vi "default zero array.vi"(7 "Array":dbl[](array[numeric]), 9 "frekans size":dbl, 10 "size":dbl, 11 "control hz array":dbl[][](array[numeric])) -> (3 "output array":dbl[][](array[numeric]))   [LabVIEW 2014]
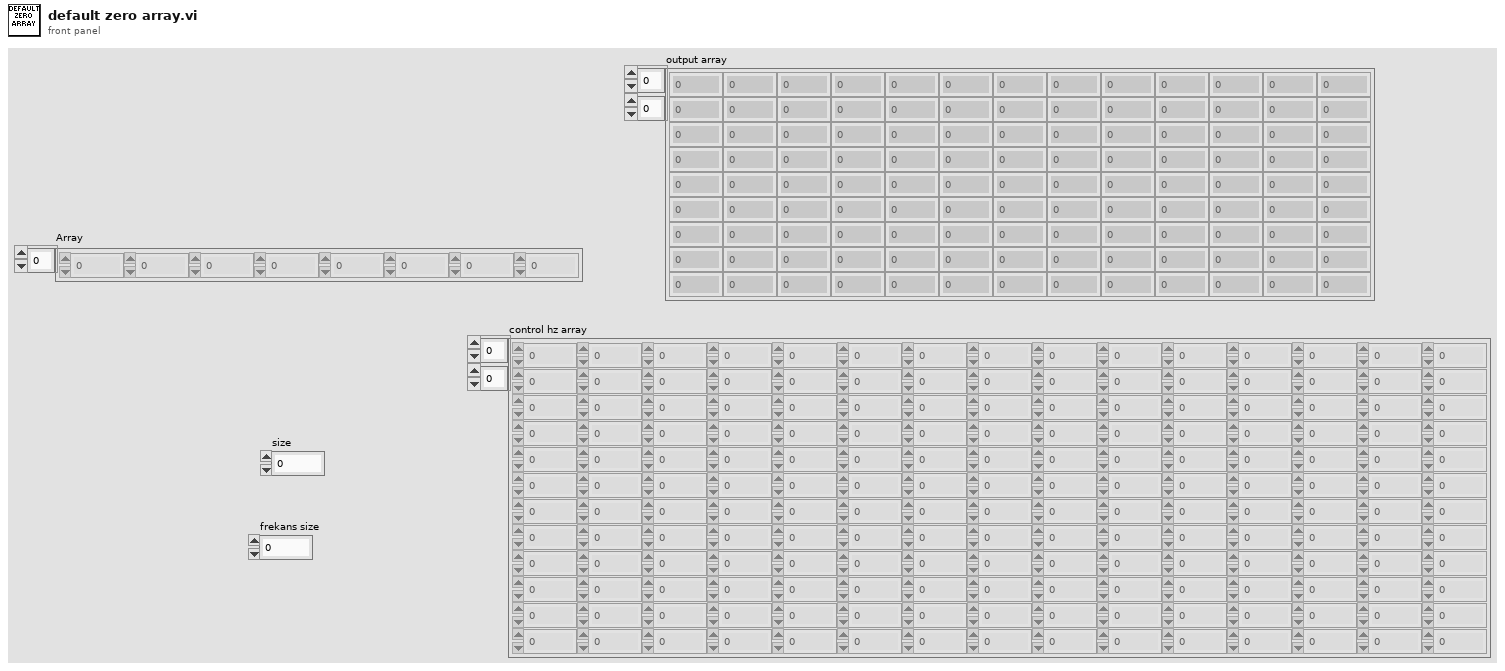
[diagram p1: front panel]
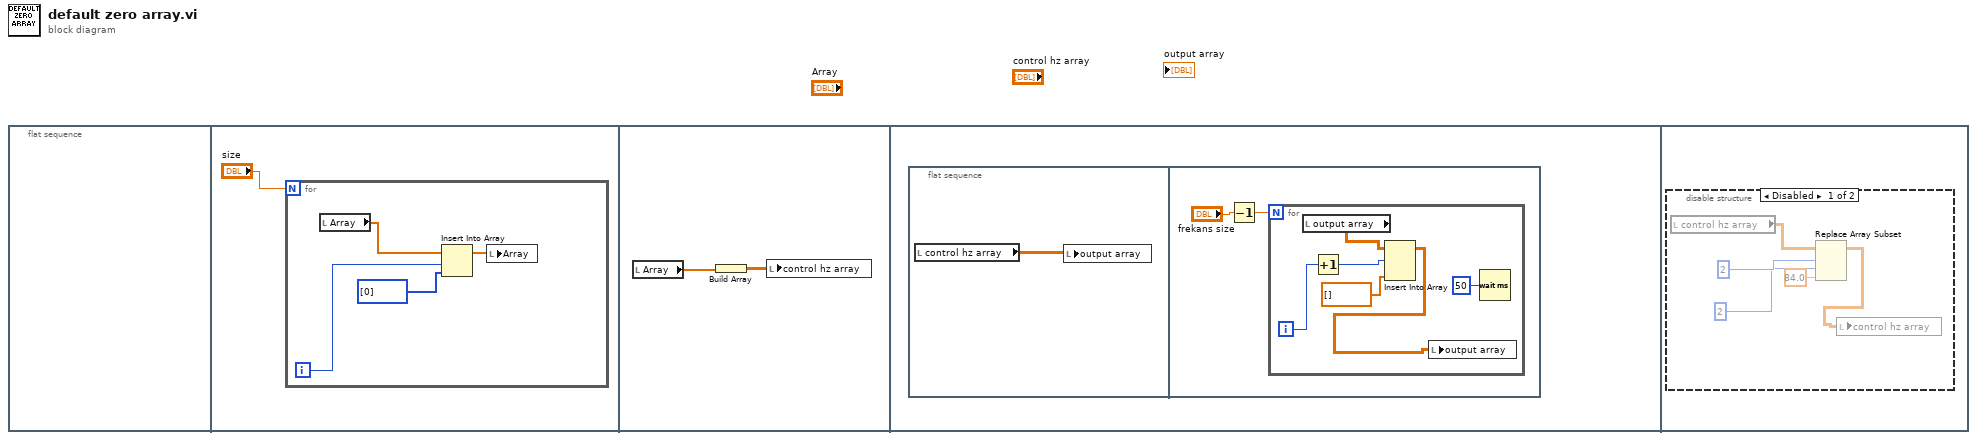
[diagram p0: block diagram]
diagram:
  n1 = flat-sequence {
    frame #0 {
    }
    frame #1 {
      n2 = for {
        N: "size" -> [_]
        i -> [w4]
        n3 = local read "Array"() -> (w5:dbl[])
        n4 = Insert Into Array(array=w5, index=w4, new element=i32[] [0]) -> (w2:dbl[])
        n5 = local write "Array"(w2) -> ()
      }
    }
    frame #2 {
      n6 = local read "Array"() -> (w7:dbl[])
      n7 = Build Array(w7) -> (w6:dbl[][])
      n8 = local write "control hz array"(w6) -> ()
    }
    frame #3 {
      n9 = flat-sequence {
        frame #0 {
          n10 = local read "control hz array"() -> (w8:dbl[][])
          n11 = local write "output array"(w8) -> ()
        }
        frame #1 {
          n12 = Decrement(x="frekans size") -> (x-1=w9:dbl)
          n13 = for {
            N: w9 -> [_]
            i -> [w15]
            n14 = local read "output array"() -> (w12:dbl[][])
            n15 = Increment(x=w15) -> (x+1=w14:i32)
            n16 = Insert Into Array(array=w12, index (row)=w14, new element=dbl[] [] ("new element/subarray")) -> (w11:dbl[][])  [unwired: 1 in]
            n17 = local write "output array"(w11) -> ()
            n18 = Wait (ms)(milliseconds to wait=u32 50) -> ()  [unwired: 1 out]
          }
        }
      }
    }
    frame #4 {
      n19 = disable-structure shown="Disabled" {
        frame Disabled {
          n20 = local read "control hz array"() -> (w21:dbl[][])
          n21 = Replace Array Subset(array=w21, new element=84.0 ("new element/subarray"), index (row)=2, index (col)=2 ("disabled index (col)")) -> (w17:dbl[][])
          n22 = local write "control hz array"(w17) -> ()
        }
        frame Enabled {
        }
      }
    }
  }
